vi "calcNewOutputs.vi"(8 "error in (no error)":errorcluster, 10 "outputData":T1 {"Step & Direction" min=-32767}, 11 "StreamingDataAlgorithm in":refnum<class "StreamingDataAlgorithm.lvclass">) -> (0 "error out":errorcluster, 2 "outputData 2":T1 {"Step & Direction" min=-32767}, 3 "StreamingDataAlgorithm out":refnum<class "StreamingDataAlgorithm.lvclass">)   [LabVIEW 2012, in "StreamingDataAlgorithm.lvclass"]
uses:
  StreamingDataAlgorithm.lvclass
  Program Files (x86)/National Instruments/LabVIEW 2012/user.lib/Common/ILC/Typedefs/OutputData.ctl
panel:
  # "DAC"
  # "DAC"
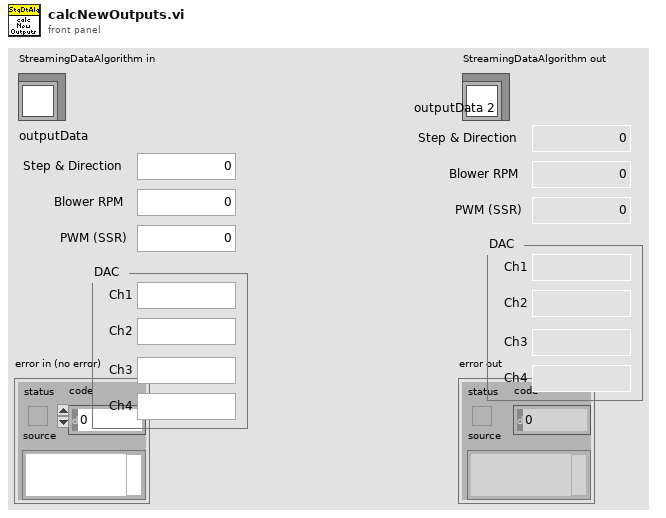
[diagram p1: front panel]
types:
  T1 = typedef "OutputData.ctl" = cluster{"Step & Direction":i16, "Blower RPM":u8, "PWM (SSR)":u8, "Ch1":u16, "Ch2":u16, "Ch3":u16, "Ch4":u16}
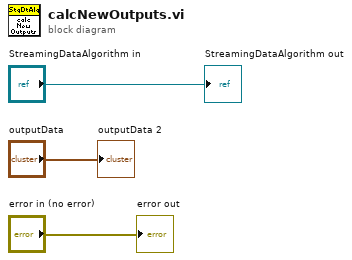
[diagram p0: block diagram]
diagram:
  "error out" <- "error in (no error)"
  "StreamingDataAlgorithm out" <- "StreamingDataAlgorithm in"
  "outputData 2" <- "outputData"
